vi "PurePursuit.vi"(0 "RobotNeededPathData":T1={"Path"=[], "MaxVel"=0.0, "MaxAccel"=0.0, "Backwards?"=FALSE, "PointSpacing"=0.0, "LookaheadDist"=0.0, "Speed/Curve"=1.8, "SlowDistanceAtEnd"=12.0, "SlowSpeed"=15.0, "MaxDeAccel"=0.0} {"SlowSpeed" format="%#_13g"; "SlowDistanceAtEnd" format="%#_13g"; "Speed/Curve" format="%#_13g"}, 1 "SensorData":T3={"LeftDistance"=0.0, "RightDistance"=0.0, "LeftVelocity"=78.75762159095939, "RightVelocity"=-76.3848555077329, "Angle"=-0.01, "Location"={11.691968699047118, 248.03471515703785}}, 3 "Trackwidth":dbl=40.0 format="%#_13g", 7 "Reset":bool, 14 "Gains":T4={"FFV"=0.0088, "FFA"=0.0017, "Vel PID"={"P"=0.02, "I"=0.0, "D"=0.0}} {"Vel PID"."D" format="%.3f"; "Vel PID"."I" format="%.3f"; "Vel PID"."P" format="%.3f"}) -> (2 "Graph":cluster{cluster{"x":dbl, "y":dbl}[]}[](graph)=[{[{"x"=20.453371592539455, "y"=249.15925394548063}, {"x"=32.451138071473615, "y"=249.2417431099791}, {"x"=44.448056211953954, "y"=249.32366698389004}, {"x"=56.441768980000354, "y"=249.4040828136747}, {"x"=68.42823711154045, "y"=249.48106130123531}, {"x"=80.3987950137465, "y"=249.55036007485356}, {"x"=92.33398719870449, "y"=249.6026243647297}, {"x"=104.19073617112089, "y"=249.61714678939316}, {"x"=115.8737280283298, "y"=249.54805321076083}, {"x"=127.17183717836993, "y"=249.29372430937337}, {"x"=137.61733743281803, "y"=248.62905317811618}, {"x"=146.1740836060984, "y"=247.05537254809167}, {"x"=150.54675993154666, "y"=243.46800813008085}, {"x"=152.39728417160754, "y"=235.46668065740275}, {"x"=152.95934006523578, "y"=225.71717171741398}, {"x"=152.6076327980232, "y"=215.7198087862704}, {"x"=151.107691158904, "y"=206.8096834259849}, {"x"=147.4595538788043, "y"=201.04671193240875}, {"x"=139.23112896790275, "y"=198.5372634006921}, {"x"=128.93601727531555, "y"=197.49649482245655}, {"x"=117.71002861894719, "y"=197.11868334076806}, {"x"=106.06838831868264, "y"=197.04007755842468}, {"x"=94.24922045605804, "y"=197.09639645188625}, {"x"=82.37229762541514, "y"=197.21330877376334}, {"x"=70.51888885096747, "y"=197.35687893558043}, {"x"=58.78593931213765, "y"=197.51094316379152}, {"x"=47.350700340581184, "y"=197.66633376164685}, {"x"=36.58889694113597, "y"=197.8147673041893}, {"x"=27.32521119491603, "y"=197.9433223158581}, {"x"=21.38307030129124, "y"=198.025824964132}]}, {[{"x"=11.691968699047118, "y"=248.03471515703785}, {"x"=23.691968516276667, "y"=248.03680955212963}]}, {[{"x"=152.95934006523578, "y"=225.71717171741398}]}, {[{"x"=26.691968699047116, "y"=248.03471515703785}, {"x"=25.95781644347442, "y"=252.66997007266207}, {"x"=23.827223614671333, "y"=256.85149394142496}, {"x"=20.508747483434213, "y"=260.16997007266207}, {"x"=16.32722361467133, "y"=262.3005629014651}, {"x"=11.69196869904712, "y"=263.03471515703785}, {"x"=7.056713783422908, "y"=262.3005629014651}, {"x"=2.875189914660023, "y"=260.16997007266207}, {"x"=-0.4432862165770928, "y"=256.85149394142496}, {"x"=-2.5738790453801847, "y"=252.66997007266207}, {"x"=-3.308031300952882, "y"=248.03471515703785}, {"x"=-2.5738790453801865, "y"=243.39946024141364}, {"x"=-0.44328621657709455, "y"=239.21793637265077}, {"x"=2.8751899146600195, "y"=235.89946024141364}, {"x"=7.056713783422905, "y"=233.76886741261055}, {"x"=11.691968699047115, "y"=233.03471515703785}, {"x"=16.327223614671325, "y"=233.76886741261055}, {"x"=20.508747483434213, "y"=235.89946024141364}, {"x"=23.82722361467133, "y"=239.21793637265074}, {"x"=25.95781644347442, "y"=243.39946024141364}, {"x"=26.691968699047116, "y"=248.03471515703785}]}, {[{"x"=16.728162111415877, "y"=242.99940064954055}, {"x"=16.48171627411582, "y"=244.55539842807914}, {"x"=15.766502597859695, "y"=245.95908430278035}, {"x"=14.652531180466154, "y"=247.0730557201739}, {"x"=13.248845305764926, "y"=247.78826939643002}, {"x"=11.692847527226334, "y"=248.03471523373008}, {"x"=10.136849748687744, "y"=247.78826939643002}, {"x"=8.733163873986515, "y"=247.0730557201739}, {"x"=7.619192456592972, "y"=245.95908430278035}, {"x"=6.903978780336848, "y"=244.55539842807914}, {"x"=6.6575329430367916, "y"=242.99940064954055}, {"x"=6.903978780336848, "y"=241.44340287100195}, {"x"=7.619192456592971, "y"=240.03971699630074}, {"x"=8.733163873986513, "y"=238.9257455789072}, {"x"=10.136849748687743, "y"=238.21053190265107}, {"x"=11.692847527226332, "y"=237.964086065351}, {"x"=13.248845305764924, "y"=238.21053190265107}, {"x"=14.652531180466152, "y"=238.9257455789072}, {"x"=15.766502597859695, "y"=240.03971699630074}, {"x"=16.48171627411582, "y"=241.44340287100195}, {"x"=16.728162111415877, "y"=242.99940064954055}]}], 4 "LeftValue":dbl=2.7501251582780792, 6 "RightValue":dbl=-2.0461251582780795, 8 "TargetVel":dbl=40.0, 10 "Done":bool)   [LabVIEW 2017]
doc: "Takes in encoder and gyro data, and a path. In real time, calculates the left and right power to send to the motors to travel the path at a specified max speed, acceleration, and lookahead distance"
uses:
  RobotNeededPathData.ctl
panel:
  in  "Max dx/dt":dbl=100.0 format="%#_13g"
  out "TargetVelGraph":dbl(graph)
  out "Waveform Chart":T2(graph)={"l"=198.87785889523798, "dx/dt"=78.75762159095939, "r"=-118.87785889523798, "dx/dt"=-76.3848555077329}
  in  "Average Vels":bool
  # "SET DEFAULTS"
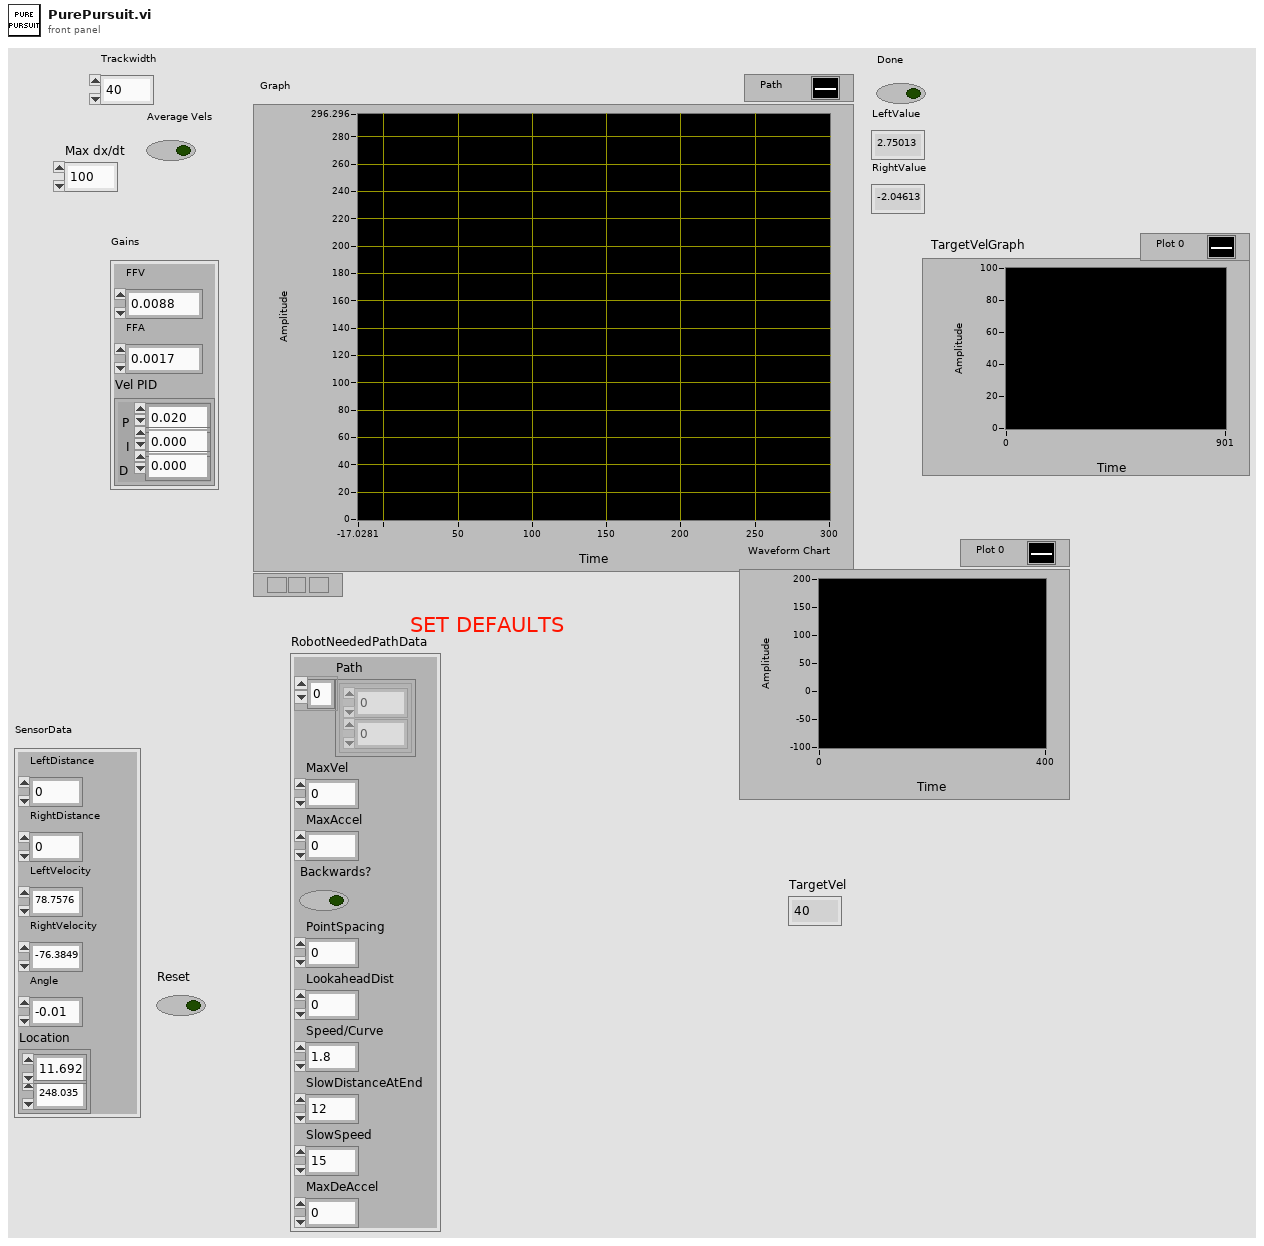
[diagram p1: front panel]
types:
  T1 = typedef "RobotNeededPathData.ctl" = cluster{"Path":cluster{dbl, dbl}[], "MaxVel":dbl, "MaxAccel":dbl, "Backwards?":bool, "PointSpacing":dbl, "LookaheadDist":dbl, "Speed/Curve":dbl, "SlowDistanceAtEnd":dbl, "SlowSpeed":dbl, "MaxDeAccel":dbl}
  T2 = cluster{"l":dbl, "dx/dt":dbl, "r":dbl, "dx/dt":dbl}
  T3 = cluster{"LeftDistance":dbl, "RightDistance":dbl, "LeftVelocity":dbl, "RightVelocity":dbl, "Angle":dbl, "Location":cluster{dbl, dbl}}
  T4 = cluster{"FFV":dbl, "FFA":dbl, "Vel PID":cluster{"P":dbl, "I":dbl, "D":dbl}}
  T5 = cluster{"Path":cluster{"x":dbl, "y":dbl}[], "Spacing":dbl, "DistancesToEnd":dbl[], "Vel":dbl[]}
  T6 = cluster{"Path":cluster{dbl, dbl}[], "PointSpacing":dbl, "DistancesToEnd":dbl[], "Vel":dbl[]}
  T7 = cluster{"l":dbl, "LeftVelocity":dbl, "r":dbl, "RightVelocity":dbl}
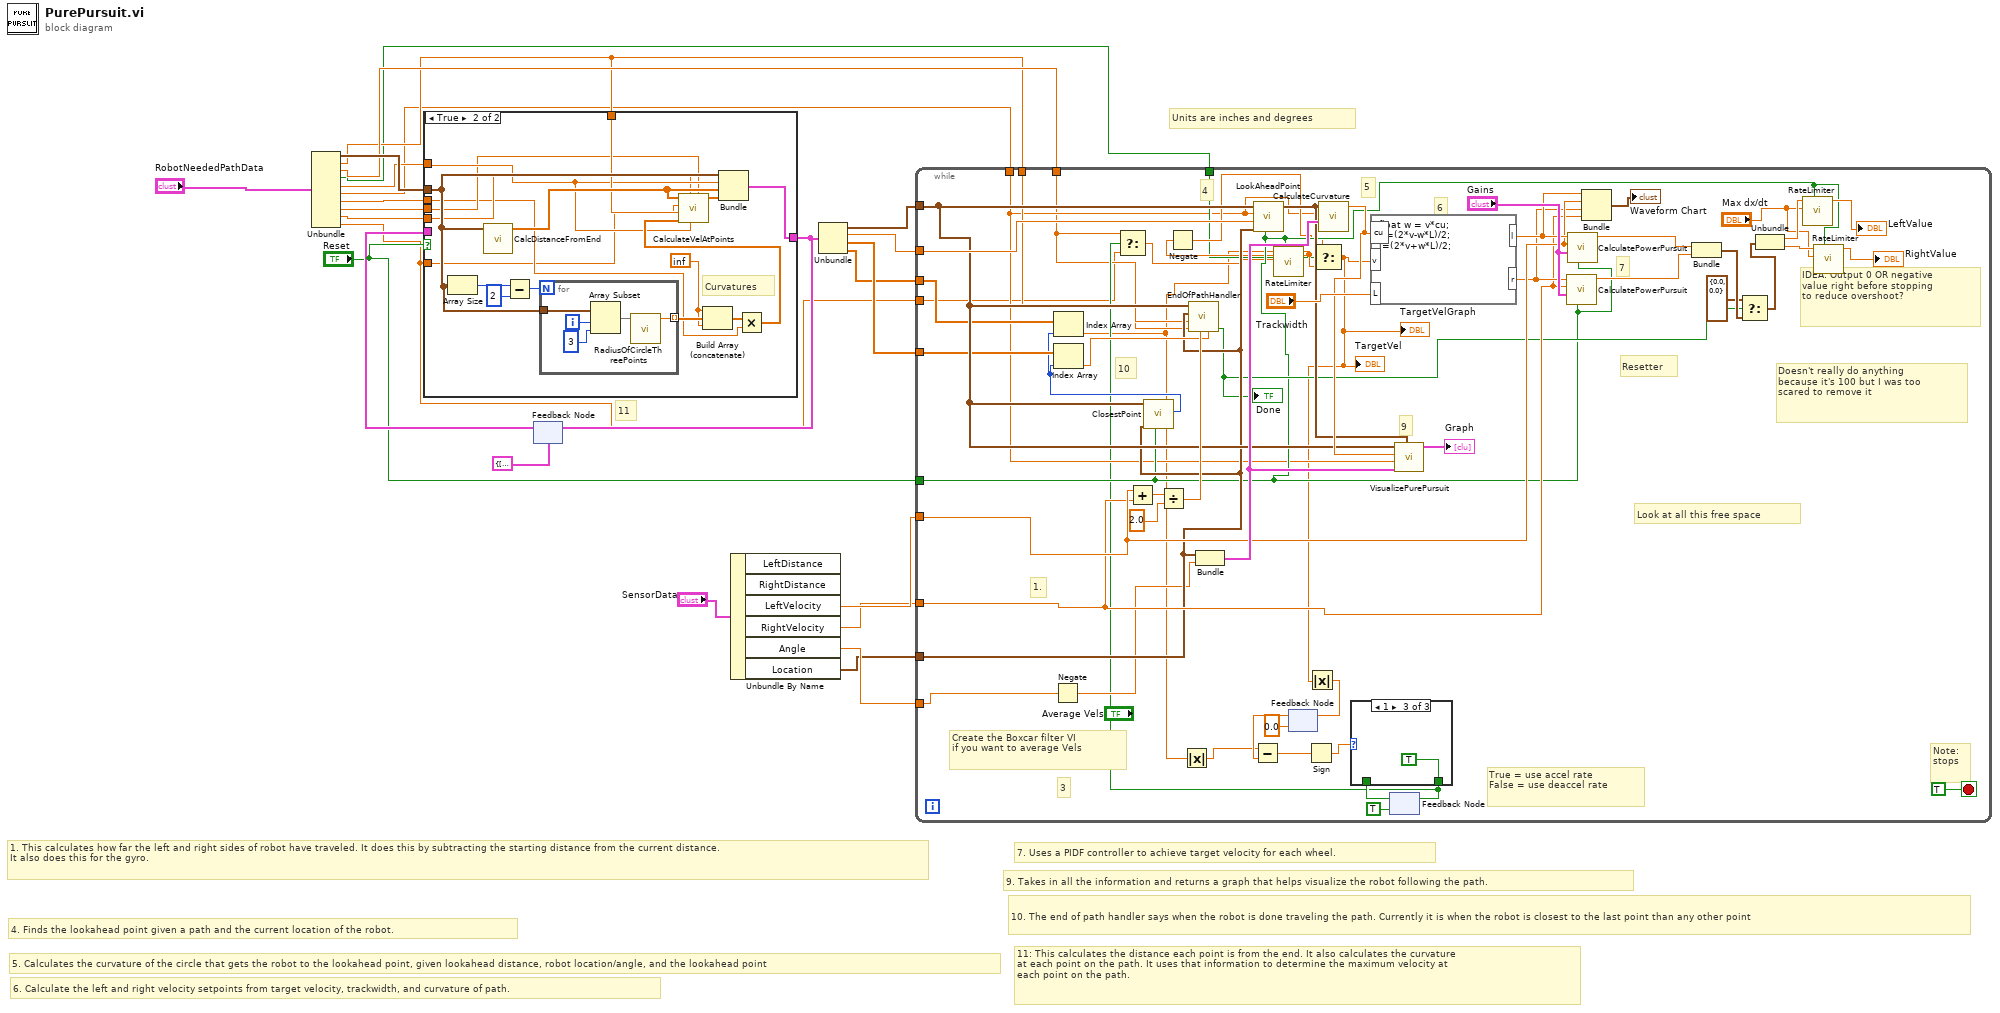
[diagram p0: block diagram]
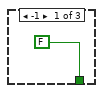
[diagram p3: hidden frame]
diagram:
  # "11: This calculates the distance each point is from the end. It also calculates the curvature\nat each point on the path. It uses that information to determine the maximum velocity at\neach point on the path."
  # "11"
  # "10. The end of path handler says when the robot is done traveling the path. Currently it is when the robot is closest to the last point than any other point"
  # "9. Takes in all the information and returns a graph that helps visualize the robot following the path."
  # "7. Uses a PIDF controller to achieve target velocity for each wheel."
  # "6. Calculate the left and right velocity setpoints from target velocity, trackwidth, and curvature of path."
  # "Units are inches and degrees"
  # "5. Calculates the curvature of the circle that gets the robot to the lookahead point, given lookahead distance, robot location/angle, and the lookahead point"
  # "4. Finds the lookahead point given a path and the current location of the robot."
  # "1. This calculates how far the left and right sides of robot have traveled. It does this by subtracting the starting distance from the current distance.\nIt also does this for the gyro."
  n1 = Unbundle("RobotNeededPathData") -> ("Path"=w10:cluster{dbl, dbl}[], "MaxVel"=w7:dbl, "MaxAccel"=w8:dbl, "Backwards?"=w6:bool, "PointSpacing"=w9:dbl, "LookaheadDist"=w5:dbl, "Speed/Curve"=w2:dbl, "SlowDistanceAtEnd"=w4:dbl, "SlowSpeed"=w3:dbl, "MaxDeAccel"=w1:dbl)
  n2 = feedback #1(T5 {"Path"=[{"x"=0.0, "y"=0.0}, {"x"=0.0, "y"=46.0}, {"x"=77.25, "y"=97.5}], "Spacing"=0.0, "DistancesToEnd"=[309.52253206522465, 306.5225388483889, 303.52254576348514, 300.5225494135135, 297.5225482930251, 294.5225431892043, 291.52253649479525, 288.5225309404311, 285.52252839669825, 282.52252922985826, 279.52253236801363, 276.5225359199274, 273.5225380077533, 270.5225374640896, 267.5225341651582, 264.5225289486152, 261.52252321975885, 258.52251843460203, 255.52251565052453, 252.52251527415513, 249.52251704698162, 246.52252022727612, 243.52252387624657, 240.5225271449837, 237.52252948071848, 234.5225307115883, 231.5225310121264, 228.5225307841412, 225.52253050297352, 222.52253057724883, 219.522531255923, 216.52253259658312, 213.5225344902357, 210.52253672481638, 207.52253906428678, 204.52254132188853, 201.52254341264756, 198.5225453787386, 195.52254738922483, 192.52254972128023, 189.5225527326013, 186.5225568345679, 183.5225624736694, 180.52257012582595, 177.52258030545136, 174.52259358906986, 171.52261065227918, 168.52263231879937, 165.52265962102405, 162.52269387257934, 159.52273675466557, 156.52279041923995, 153.52285761342083, 150.52294183093122, 147.52304749810799, 144.52318020416902, 141.5233469881785, 138.52355669860665, 135.52382044572104, 132.52415217017628, 129.52456938475245, 126.52509392552396, 123.52575388229783, 120.52658224756205, 117.52762599636499, 114.52893466674816, 111.5305811433295, 108.53265099247815, 105.5352499693053, 102.53851522329074, 99.54261858949184, 96.54777258499563, 93.55424339621041, 90.56236601643654, 87.57255952674781, 84.58534501572932, 81.60137180227034, 78.62143961905741, 75.64655567097594, 72.6779255489502, 69.71706974165639, 66.76578984976493, 63.82625595622302, 60.90103565379168, 57.99306437227732, 55.10557379235981, 52.24189700353533, 49.40502603383819, 46.59675379579783, 43.81612021857386, 41.056705992040605, 38.30212773163372, 35.53590323835957, 32.752089130751756, 29.950811925036337, 27.135602619179224, 24.311917874683846, 21.486403150766286, 18.666614193530503, 15.861028930660632, 13.07925664424869, 10.33239795871144, 7.633538890247935, 4.998382632368401, 2.4460384085185156, 0.0], "Vel"=[309.52253206522465, 306.5225388483889, 303.52254576348514, 300.5225494135135, 297.5225482930251, 294.5225431892043, 291.52253649479525, 288.5225309404311, 285.52252839669825, 282.52252922985826, 279.52253236801363, 276.5225359199274, 273.5225380077533, 270.5225374640896, 267.5225341651582, 264.5225289486152, 261.52252321975885, 258.52251843460203, 255.52251565052453, 252.52251527415513, 249.52251704698162, 246.52252022727612, 243.52252387624657, 240.5225271449837, 237.52252948071848, 234.5225307115883, 231.5225310121264, 228.5225307841412, 225.52253050297352, 222.52253057724883, 219.522531255923, 216.52253259658312, 213.5225344902357, 210.52253672481638, 207.52253906428678, 204.52254132188853, 201.52254341264756, 198.5225453787386, 195.52254738922483, 192.52254972128023, 189.5225527326013, 186.5225568345679, 183.5225624736694, 180.52257012582595, 177.52258030545136, 174.52259358906986, 171.52261065227918, 168.52263231879937, 165.52265962102405, 162.52269387257934, 159.52273675466557, 156.52279041923995, 153.52285761342083, 150.52294183093122, 147.52304749810799, 144.52318020416902, 141.5233469881785, 138.52355669860665, 135.52382044572104, 132.52415217017628, 129.52456938475245, 126.52509392552396, 123.52575388229783, 120.52658224756205, 117.52762599636499, 114.52893466674816, 111.5305811433295, 108.53265099247815, 105.5352499693053, 102.53851522329074, 99.54261858949184, 96.54777258499563, 93.55424339621041, 90.56236601643654, 87.57255952674781, 84.58534501572932, 81.60137180227034, 78.62143961905741, 75.64655567097594, 72.6779255489502, 69.71706974165639, 66.76578984976493, 63.82625595622302, 60.90103565379168, 57.99306437227732, 55.10557379235981, 52.24189700353533, 49.40502603383819, 46.59675379579783, 43.81612021857386, 41.056705992040605, 38.30212773163372, 35.53590323835957, 32.752089130751756, 29.950811925036337, 27.135602619179224, 24.311917874683846, 21.486403150766286, 18.666614193530503, 15.861028930660632, 13.07925664424869, 10.33239795871144, 7.633538890247935, 4.998382632368401, 2.4460384085185156, 0.0]} ("PathData")) -> (w14:T5)
  n3 = case shown="True" "Reset" {
    tunnel: [w25 w41] -> w13
    tunnel: w14 -> [w25 _]
    tunnel: w7 -> [_ w32]
    tunnel: w10 -> [_ w34]
    tunnel: w9 -> [_ w30]
    tunnel: w4 -> [_ w29]
    tunnel: w3 -> [_ w28]
    tunnel: w2 -> [_ w27]
    tunnel: w1 -> [_ w26]
    frame False {
    }
    frame True {
      w36 = inf
      # "Curvatures"
      n4 = Array Size(array=w34) -> (size(s)=w37:i32)
      n5 = call "CalcDistanceFromEnd.vi"("Path"=w34) -> ("DistancesToEnd"=w33:dbl[])  [unwired: 10 in]
      n6 = Subtract(x=w37, y=2) -> (x-y=w38:i32)
      n7 = for {
        N: w38 -> [_]
        tunnel: w34 -> [w47]
        tunnel: [w43] -> w39 mode=indexing
        i -> [w46]
        n8 = Array Subset(array=w47, index=w46, length=3) -> (w44:cluster{dbl, dbl}[])
        n9 = call "RadiusOfCircleThreePoints.vi"("Points"=w44) -> ("R"=w43:dbl)  [unwired: 10 in]
      }
      n10 = Build Array (concatenate)(w36, w39, w36) -> (w40:dbl[])
      n11 = Multiply(x=w40, y=w27) -> (x*y=w31:dbl[])
      n12 = call "CalculateVelAtPoints.vi"("DistanceSlowAtEnd"=w29, "Spacing"=w30, "SlowSpeed"=w28, "MaxVels"=w31, "MaxVel"=w32, "MaxAccel"=w26, "DistancesToEnd"=w33) -> ("Vel"=w42:dbl[])  [unwired: 4 in]
      n13 = Bundle("Path"=w34, "PointSpacing"=w30, "DistancesToEnd"=w33, "Vel"=w42) -> (w41:T6)  [unwired: 1 in]
    }
  }
  n14 = feedback-in #1(w13) -> ()
  n15 = Unbundle By Name("SensorData") -> ("LeftVelocity"=w23:dbl, "RightVelocity"=w22:dbl, "Angle"=w17:dbl, "Location"=w16:cluster{dbl, dbl})  [unwired: 2 out]
  n16 = Unbundle(w13) -> ("Path"=w21:cluster{"x":dbl, "y":dbl}[], "PointSpacing"=w20:dbl, "DistancesToEnd"=w19:dbl[], "Vel"=w18:dbl[])
  n17 = while {
    tunnel: w21 -> [w85]
    tunnel: w20 -> [w102]
    tunnel: w23 -> [w88]
    tunnel: w22 -> [w86]
    tunnel: w17 -> [w74]
    tunnel: w19 -> [w83]
    tunnel: w18 -> [w81]
    tunnel: w16 -> [w76]
    tunnel: w8 -> [w55]
    tunnel: w7 -> [w75]
    tunnel: "Reset" -> [w66]
    tunnel: w6 -> [w63]
    tunnel: w5 -> [w62]
    tunnel: w1 -> [w48]
    stop <- TRUE stop-if-true
    # "True = use accel rate\nFalse = use deaccel rate"
    # "Doesn't really do anything\nbecause it's 100 but I was too\nscared to remove it"
    # "Create the Boxcar filter VI\nif you want to average Vels"
    # "Look at all this free space"
    # "Note:\nstops"
    # "IDEA: Output 0 OR negative\nvalue right before stopping\nto reduce overshoot?"
    # "10"
    # "9"
    # "7"
    # "6"
    # "5"
    # "4"
    # "3"
    # "1."
    # "Resetter"
    n18 = Negate(x=w74) -> (-x=w73:dbl)
    n19 = Add(x=w88, y=w86) -> (x+y=w94:dbl)
    n20 = call "ClosestPoint.vi"("Reset"=w66, "Robot"=w76, "Path"=w85) -> ("ClosestIndex"=w80:i32)  [unwired: 7 in, 1 out]
    n21 = Index Array(array=w81, index=w80) -> (element=w54:dbl)
    n22 = Index Array(array=w83, index=w80) -> (element=w82:dbl)
    n23 = Divide(x=w94, y=2.0) -> (x/y=w92:dbl)
    n24 = Absolute Value(x=w54) -> (abs(x)=w50:dbl)
    n25 = call "EndOfPathHandler.vi"("DistanceToEnd"=w82, "CurrentVel"=w92, "MaxAccel"=w55, "MaxVel"=w75, "RobotLocation"=w76, "Path"=w85) -> ("Done"=w72:bool)  [unwired: 2 in, 3 out]
    "Done" <- w72
    n26 = Bundle("Location"=w76, w73) -> (w98:cluster{"Location":cluster{dbl, dbl}, dbl})  [unwired: 1 in]
    n27 = call "LookAheadPoint.vi"("Reset"=w66, "Robot"=w76, "Spacing"=w102, "LookAhead"=w62, "Path"=w85) -> ("Point"=w97:cluster{"x":dbl, "y":dbl})  [unwired: 5 in, 1 out]
    n28 = feedback #2(0.0) -> (w51:dbl)
    n29 = Subtract(x=w50, y=w51) -> (x-y=w61:dbl)
    n30 = Sign(1:w61) -> (0:w60:dbl)
    n31 = call "CalculateCurvature.vi"("Robot"=w98, "Lookahead"=w62, "Point"=w97) -> ("Curvature"=w99:dbl)  [unwired: 8 in]
    n32 = feedback #3(TRUE) -> (w59:bool)
    n33 = case shown="1" w60 {
      tunnel: [FALSE w104 TRUE] -> w57
      tunnel: w59 -> [_ w104 _]
      frame -1 {
      }
      frame 0, Default {
      }
      frame 1 {
      }
    }
    n34 = Select(t=w55, s=w57, f=w48) -> (s? t:f=w56:dbl)
    n35 = call "RateLimiter.vi"("Reset"=w66, "Max dx/dt"=w56, "Input"=w54) -> ("Output"=w65:dbl)  [unwired: 8 in]
    n36 = Negate(x=w65) -> (-x=w64:dbl)
    n37 = Select(t=w64, s=w63, f=w65) -> (s? t:f=w53:dbl)
    "TargetVel" <- w53
    "TargetVelGraph" <- w53
    n38 = Absolute Value(x=w53) -> (abs(x)=w52:dbl)
    n39 = feedback-in #2(w52) -> ()
    n40 = formula code="float w = v*cu;\nr =(2*v-w*L)/2;\nl=(2*v+w*L)/2;"("L"="Trackwidth", "cu"=w99, "v"=w53) -> ("r"=w87:dbl, "l"=w90:dbl)
    n41 = feedback-in #3(w57) -> ()
    n42 = call "VisualizePurePursuit.vi"("Lookahead Point"=w97, "Robot"=w98, "Lookahead"=w62, "Curvature"=w99, "Path"=w85) -> ("Graph"=→"Graph":cluster{cluster{"x":dbl, "y":dbl}[]}[])  [unwired: 6 in]
    n43 = call "CalculatePowerPursuit.vi"("Reset"=w66, "Gains"="Gains", "Vel"=w86, "Target Vel"=w87) -> ("Power"=w95:dbl)  [unwired: 7 in]
    n44 = call "CalculatePowerPursuit.vi"("Reset"=w66, "Gains"="Gains", "Vel"=w88, "Target Vel"=w90) -> ("Power"=w96:dbl)  [unwired: 7 in]
    n45 = Bundle("l"=w90, "LeftVelocity"=w88, "r"=w87, "RightVelocity"=w86) -> (→"Waveform Chart":T7)  [unwired: 1 in]
    n46 = Bundle("Power"=w96, "Power"=w95) -> (w79:cluster{"Power":dbl, "Power":dbl})  [unwired: 1 in]
    n47 = Select(t=cluster{"Power":dbl, "Power":dbl} {"Power"=0.0, "Power"=0.0}, s=w72, f=w79) -> (s? t:f=w77:cluster{"Power":dbl, "Power":dbl})
    n48 = Unbundle(w77) -> ("Power"=w71:dbl, "Power"=w70:dbl)
    n49 = call "RateLimiter.vi"("Reset"=w66, "Max dx/dt"="Max dx/dt", "Input"=w71) -> ("Output"=→"LeftValue":dbl)  [unwired: 8 in]
    n50 = call "RateLimiter.vi"("Reset"=w66, "Max dx/dt"="Max dx/dt", "Input"=w70) -> ("Output"=→"RightValue":dbl)  [unwired: 8 in]
  }
